vi "gentec-SOLO-PE.Statistics.vi"(8 "error in (no error)":errorcluster, 11 "VISA Refnum in":refnum<visa-resource-name>) -> (0 "error out":errorcluster, 1 "Statistic Data":T1 {"Uncorrected Value" format="%.6f"; "Rep Rate" format="%.2f"; "Average Power" format="%.6f"; "PTP Stability" format="%.6f"; "RMS Stability" format="%.6f"; "Standard Deviation" format="%.6f"; "Average" format="%.6f"; "Minimum" format="%.6f"; "Maximum" format="%.6f"; "Current Value" format="%.6f"}, 2 "Error":string, 3 "VISA Refnum out":refnum<visa-resource-name>, 4 "Timeout":bool)   [LabVIEW 2014, in "gentec-SOLO-PE - Driver.lvlib"]
doc: "This VI reads out the statistic data."
uses:
  gentec-SOLO-PE - Driver.lvlib
  Type Defs/gentec-SOLO-PE.Statistics Data.ctl
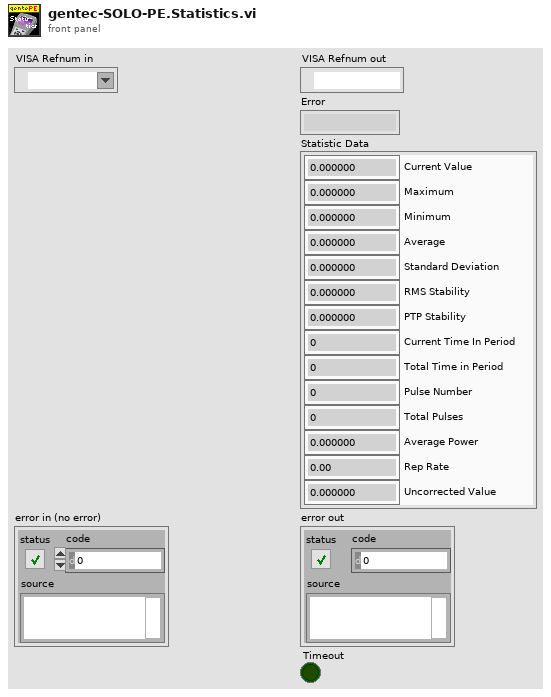
[diagram p1: front panel]
types:
  T1 = typedef "gentec-SOLO-PE - Driver.lvlib/gentec-SOLO-PE.Statistics Data.ctl" = cluster{"Current Value":dbl, "Maximum":dbl, "Minimum":dbl, "Average":dbl, "Standard Deviation":dbl, "RMS Stability":dbl, "PTP Stability":dbl, "Current Time In Period":u32, "Total Time in Period":u32, "Pulse Number":u32, "Total Pulses":u32, "Average Power":dbl, "Rep Rate":dbl, "Uncorrected Value":dbl}
  T2 = cluster{"Return Parameters[0]":u32, "Return Parameters[1]":u32, "Return Parameters[2]":u32, "Return Parameters[3]":u32, "Return Parameters[4]":u32, "Return Parameters[5]":u32, "Return Parameters[6]":u32, "Return Parameters[7]":u32, "Return Parameters[8]":u32, "Return Parameters[9]":u32, "Return Parameters[10]":u32, "Return Parameters[11]":u32, "Return Parameters[12]":u32, "Return Parameters[13]":u32, "Return Parameters[14]":u32, "Return Parameters[15]":u32, "Return Parameters[16]":u32, "Return Parameters[17]":u32, "Return Parameters[18]":u32, "Return Parameters[19]":u32, "Return Parameters[20]":u32, "Return Parameters[21]":u32}
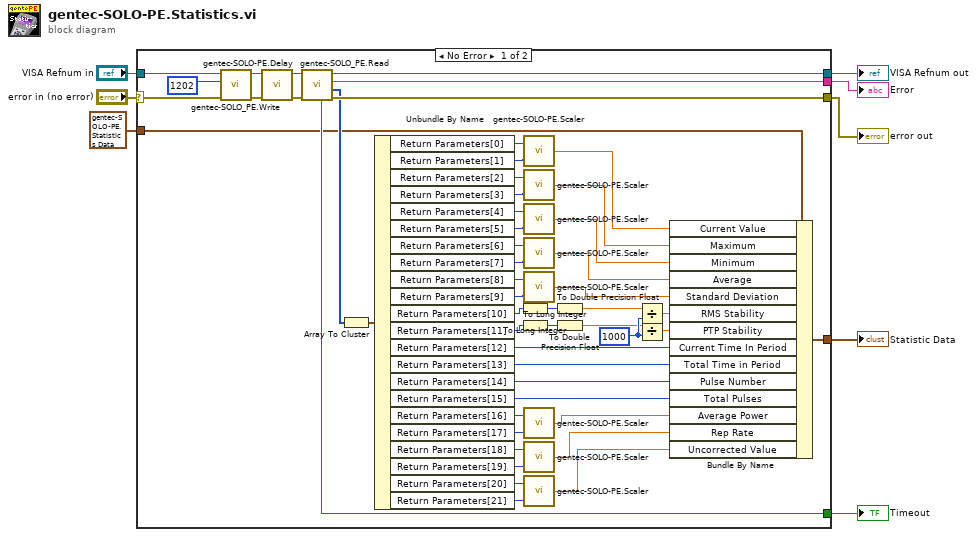
[diagram p0: block diagram]
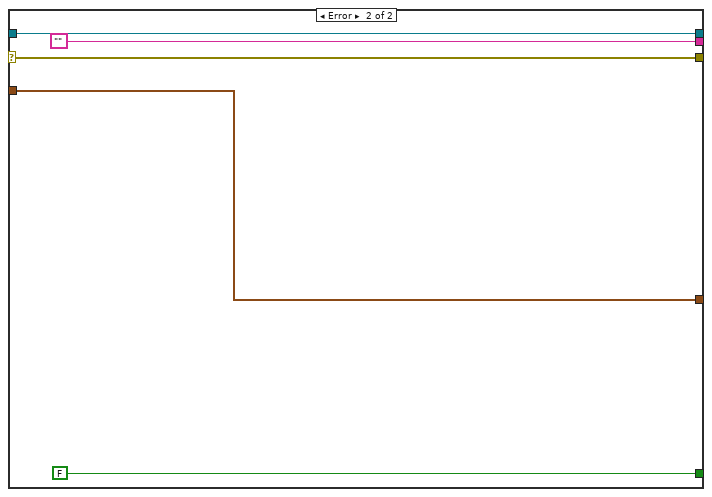
[diagram p2: hidden frame]
diagram:
  n1 = case shown="No Error" "error in (no error)" {
    selector: "error in (no error)" -> [w52 w64]
    tunnel: [w50 w64] -> w8
    tunnel: [w60 w65] -> w7
    tunnel: [w51 ""] -> w3
    tunnel: [w59 FALSE ("Timeout")] -> w6
    tunnel: "VISA Refnum in" -> [w54 w65]
    tunnel: T1 {"Current Value"=0.0, "Maximum"=0.0, "Minimum"=0.0, "Average"=0.0, "Standard Deviation"=0.0, "RMS Stability"=0.0, "PTP Stability"=0.0, "Current Time In Period"=0, "Total Time in Period"=0, "Pulse Number"=0, "Total Pulses"=0, "Average Power"=0.0, "Rep Rate"=0.0, "Uncorrected Value"=0.0} ("Statistic Data") -> [w10 w61]
    tunnel: [w9 w61] -> w1
    frame No Error {
      w45 = 1000
      n2 = call "gentec-SOLO_PE.Write.vi"("error in (no error)"=w52, "Command Handle"=u16 1202, "VISA Refnum in"=w54) -> ("error out"=w57:errorcluster, "VISA Refnum out"=w55:refnum<visa-resource-name>)  [unwired: 7 in]
      n3 = call "gentec-SOLO-PE.Delay.vi"("error in (no error)"=w57, "VISA resource In"=w55) -> ("error out"=w58:errorcluster, "VISA resource Out"=w56:refnum<visa-resource-name>)  [unwired: 4 in]
      n4 = call "gentec-SOLO_PE.Read.vi"("error in (no error)"=w58, "VISA Refnum in"=w56) -> ("error out"=w50:errorcluster, "Return Parameters"=w11:u32[], "Error"=w51:string, "VISA Refnum out"=w60:refnum<visa-resource-name>, "Timeout"=w59:bool)  [unwired: 5 in]
      n5 = Array To Cluster(array=w11) -> (cluster=w49:T2)
      n6 = Unbundle By Name(w49) -> ("Return Parameters[0]"=w35:u32, "Return Parameters[1]"=w33:u32, "Return Parameters[2]"=w31:u32, "Return Parameters[3]"=w32:u32, "Return Parameters[4]"=w27:u32, "Return Parameters[5]"=w28:u32, "Return Parameters[6]"=w24:u32, "Return Parameters[7]"=w25:u32, "Return Parameters[8]"=w21:u32, "Return Parameters[9]"=w22:u32, "Return Parameters[10]"=w43:u32, "Return Parameters[11]"=w42:u32, "Return Parameters[12]"=w39:u32, "Return Parameters[13]"=w38:u32, "Return Parameters[14]"=w37:u32, "Return Parameters[15]"=w36:u32, "Return Parameters[16]"=w19:u32, "Return Parameters[17]"=w18:u32, "Return Parameters[18]"=w16:u32, "Return Parameters[19]"=w15:u32, "Return Parameters[20]"=w12:u32, "Return Parameters[21]"=w13:u32)
      n7 = To Long Integer(number=w43) -> (32bit integer=w48:i32)
      n8 = To Long Integer(number=w42) -> (32bit integer=w47:i32)
      n9 = call "gentec-SOLO-PE.Scaler.vi"("Scaler"=w33, "Value"=w35) -> ("Scaled Value"=w34:dbl)
      n10 = call "gentec-SOLO-PE.Scaler.vi"("Scaler"=w32, "Value"=w31) -> ("Scaled Value"=w30:dbl)
      n11 = call "gentec-SOLO-PE.Scaler.vi"("Scaler"=w28, "Value"=w27) -> ("Scaled Value"=w29:dbl)
      n12 = call "gentec-SOLO-PE.Scaler.vi"("Scaler"=w25, "Value"=w24) -> ("Scaled Value"=w26:dbl)
      n13 = call "gentec-SOLO-PE.Scaler.vi"("Scaler"=w22, "Value"=w21) -> ("Scaled Value"=w23:dbl)
      n14 = call "gentec-SOLO-PE.Scaler.vi"("Scaler"=w18, "Value"=w19) -> ("Scaled Value"=w20:dbl)
      n15 = call "gentec-SOLO-PE.Scaler.vi"("Scaler"=w15, "Value"=w16) -> ("Scaled Value"=w17:dbl)
      n16 = call "gentec-SOLO-PE.Scaler.vi"("Scaler"=w13, "Value"=w12) -> ("Scaled Value"=w14:dbl)
      n17 = To Double Precision Float(number=w48) -> (double precision float=w46:dbl)
      n18 = To Double Precision Float(number=w47) -> (double precision float=w44:dbl)
      n19 = Divide(x=w46, y=w45) -> (x/y=w41:dbl)
      n20 = Divide(x=w44, y=w45) -> (x/y=w40:dbl)
      n21 = Bundle By Name(cluster=w10, "Current Value"=w34, "Maximum"=w30, "Minimum"=w29, "Average"=w26, "Standard Deviation"=w23, "RMS Stability"=w41, "PTP Stability"=w40, "Current Time In Period"=w39, "Total Time in Period"=w38, "Pulse Number"=w37, "Total Pulses"=w36, "Average Power"=w20, "Rep Rate"=w17, "Uncorrected Value"=w14) -> (w9:T1)
    }
    frame Error {
    }
  }
  "error out" <- w8
  "VISA Refnum out" <- w7
  "Error" <- w3
  "Timeout" <- w6
  "Statistic Data" <- w1
